vi "PXI-Is Any Task 16-bit.vi"(7 "Task Array":T1[](array[typedef]), 11 "error in (no error)":errorcluster) -> (8 "Any 16-bit task?":bool, 15 "error out":errorcluster)   [LabVIEW 2020]
uses:
  AODO/Typedefs/AODO-Task Specification.ctl
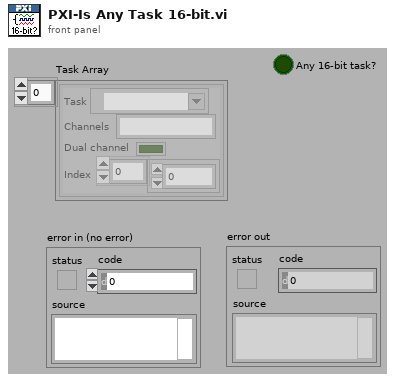
[diagram p1: front panel]
types:
  T1 = typedef "AODO-Task Specification.ctl" = cluster{"Task":refnum<k21>, "Channels":string, "Dual channel":bool, "Index":i32[]}
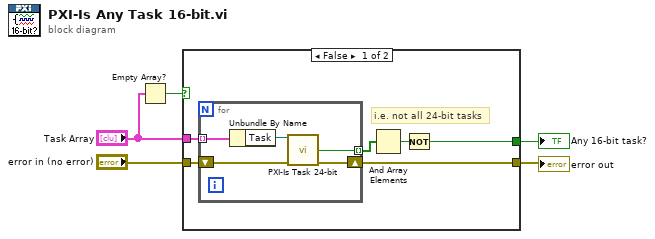
[diagram p0: block diagram]
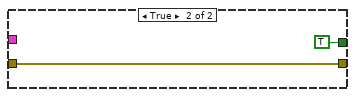
[diagram p2: hidden frame]
diagram:
  n1 = Empty Array?(array="Task Array") -> (empty?=w2:bool)
  n2 = case shown="False" w2 {
    tunnel: "error in (no error)" -> [w11 w18]
    tunnel: [w9 w18] -> w4
    tunnel: [w8 TRUE] -> w3
    tunnel: "Task Array" -> [w6 _]
    frame False {
      # "i.e. not all 24-bit tasks"
      n3 = for {
        tunnel: w6 -> [w16] mode=indexing
        shift-right: [w14] -> w9
        shift-left: w11 -> [w15]
        tunnel: [w13] -> w7 mode=indexing
        n4 = Unbundle By Name(w16) -> ("Task"=w12:refnum<k21>)
        n5 = call "PXI-Is Task 24-bit.vi"("task"=w12, "error in (no error)"=w15) -> ("is 24bit?"=w13:bool, "error out"=w14:errorcluster)  [unwired: 8 in, 4 out]
      }
      n6 = And Array Elements(Boolean array=w7) -> (logical AND=w10:bool)
      n7 = Not(x=w10) -> (.not. x?=w8:bool)
    }
    frame True {
    }
  }
  "error out" <- w4
  "Any 16-bit task?" <- w3
